vi "check_is_empty.vi"(1 "Channels":tag[](array[tag])) -> (0 "Has Empty?":bool)   [LabVIEW 2015]
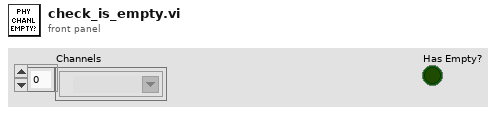
[diagram p1: front panel]
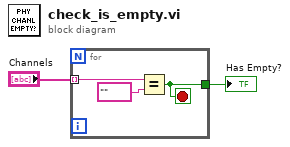
[diagram p0: block diagram]
diagram:
  n1 = for {
    tunnel: "Channels" -> [w5] mode=indexing
    tunnel: [w4] -> w1
    stop <- w4 stop-if-true
    n2 = Equal?(x=w5, y=tag "" ("DAQmx Physical Channel")) -> (x = y?=w4:bool)
  }
  "Has Empty?" <- w1
